vi "Aux2 FPGA.vi"() -> ()   [LabVIEW 2020]
uses:
  <vilib>/LabVIEW Targets/FPGA/cRIO/shared/nicrio_ModuleControls/nicrio_cRIO-9467_Latitude.ctl
  <vilib>/LabVIEW Targets/FPGA/cRIO/shared/nicrio_ModuleControls/nicrio_cRIO-9467_Longitude.ctl
  <vilib>/LabVIEW Targets/FPGA/cRIO/shared/nicrio_ModuleControls/nicrio_cRIO-9467_Altitude.ctl
  <vilib>/rvi/Emulation/niFpgaGetClockAttributes.vi
  <vilib>/rvi/Emulation/niFpgaSctlEmulationGetInTimedLoop.vi
  <vilib>/rvi/Emulation/niFpgaEmulationReportErrorSimple.vi
  subVIs/Front Panel Globals.vi
  <vilib>/rvi/interface/RandomDataEmulation/niFpgaRandomDataHandleErrors.vi
  <vilib>/rvi/Emulation/niFpgaCriticalErrorInLSC.vi
  <vilib>/rvi/Emulation/niFpgaProcessEmulError.vi
  <vilib>/rvi/DataTransferAndStorage/Container/XNode/niFpgaContainer.xnode
  <vilib>/rvi/interface/RandomDataEmulation/nirviRandomDataFpgaReadWriteTemplate.vi
panel:
  out "GPS Self-Survey Complete":bool
  out "GPS Firmware Version":u32
  out "GPS Vendor ID":u16
  out "GPS Altitude (m)":T1 format="%.2f"
  out "GPS Longitude (°)":T2 format="%.6g"
  out "GPS Latitude (°)":T3 format="%.6f"
  out "GPS Serial Number":u32
  out "GPS Time Lock":bool
  out "GPS Time (ns)":u64
  out "GPS Status":T4(ring)
  out "GPS Time Offset":i32
  out "GPS Antenna Status":T5(ring)
  out "GPS Satelites Available":u8
  out "GPS UTC Offset":i8
  out "GPS UTC Offset Valid":bool
  out "Analog Acquisition Looprate":sgl
  in  "Enable Analog Acquisition":bool
  out "Analog Channel Count":i32
  in  "Analog Acquisition Rate":sgl=10000.0
  in  "FPGA USER1 LED":bool
  out "Watchdog Whack Count":u32
  in  "FPGA System Reset":bool
  out "Watchdog ms Since Whack":u32
  in  "Watchdog Whack":bool
  in  "Watchdog Timeout (ms)":u32=3600000
  in  "Watchdog Enable":bool
  out "FPGA Nanosecond Counter":i64
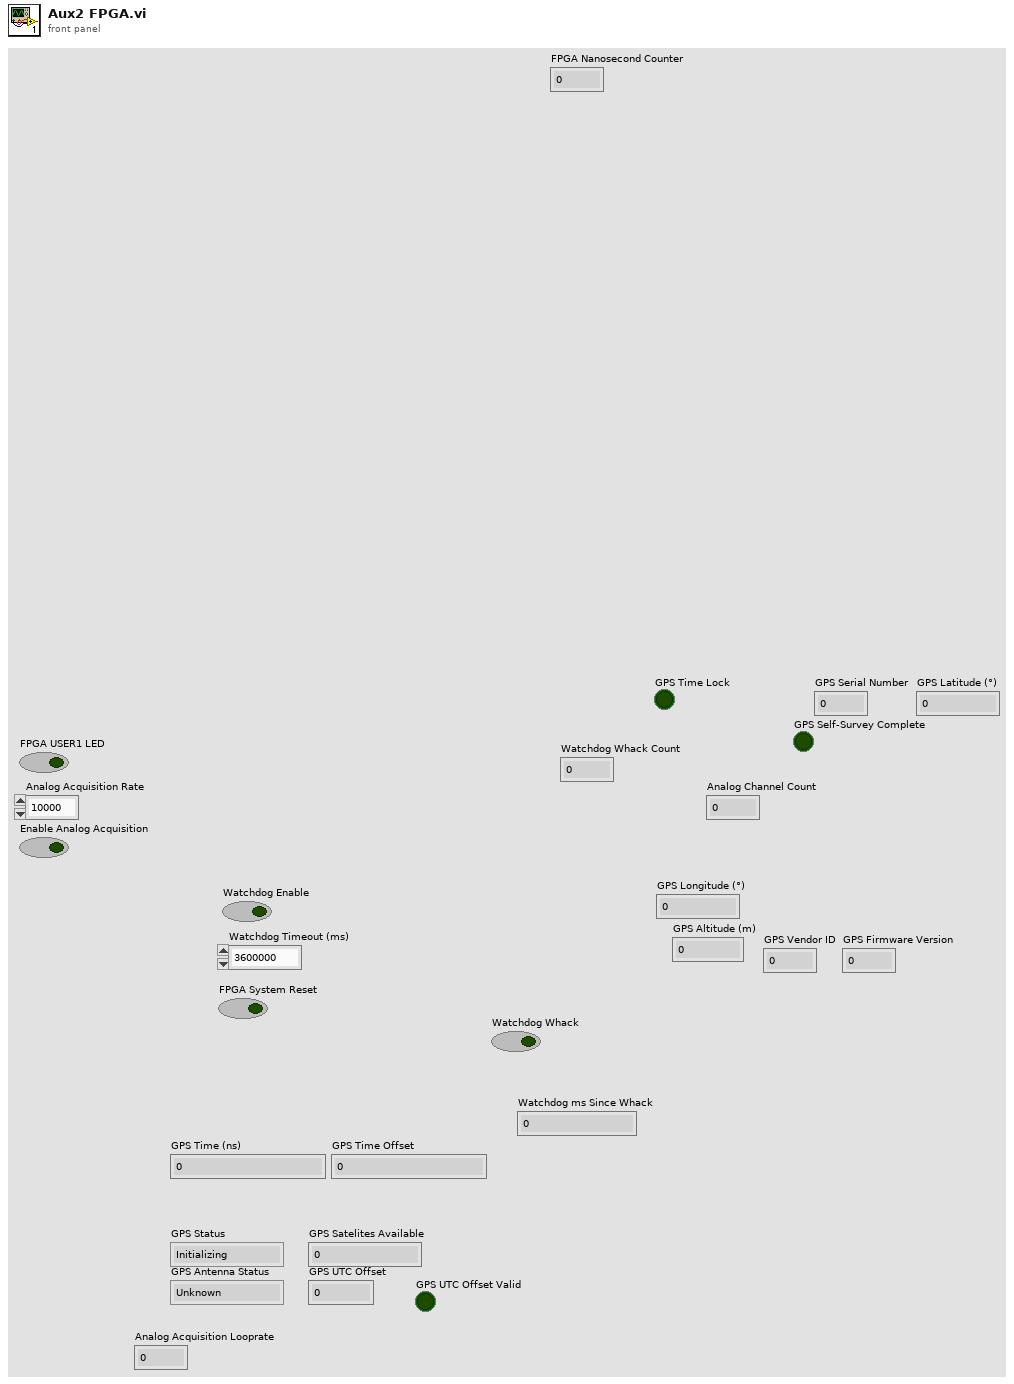
[diagram p1: front panel]
types:
  T1 = typedef "nicrio_cRIO-9467_Altitude.ctl" = fxp<+/-,24,17>
  T2 = typedef "nicrio_cRIO-9467_Longitude.ctl" = fxp<+/-,29,9>
  T3 = typedef "nicrio_cRIO-9467_Latitude.ctl" = fxp<+/-,28,8>
  T4 = enum8{"Initializing", "Normal", "Unable to get fix"}
  T5 = enum8{"Unknown", "Normal", "Absent", "Overcurrent"}
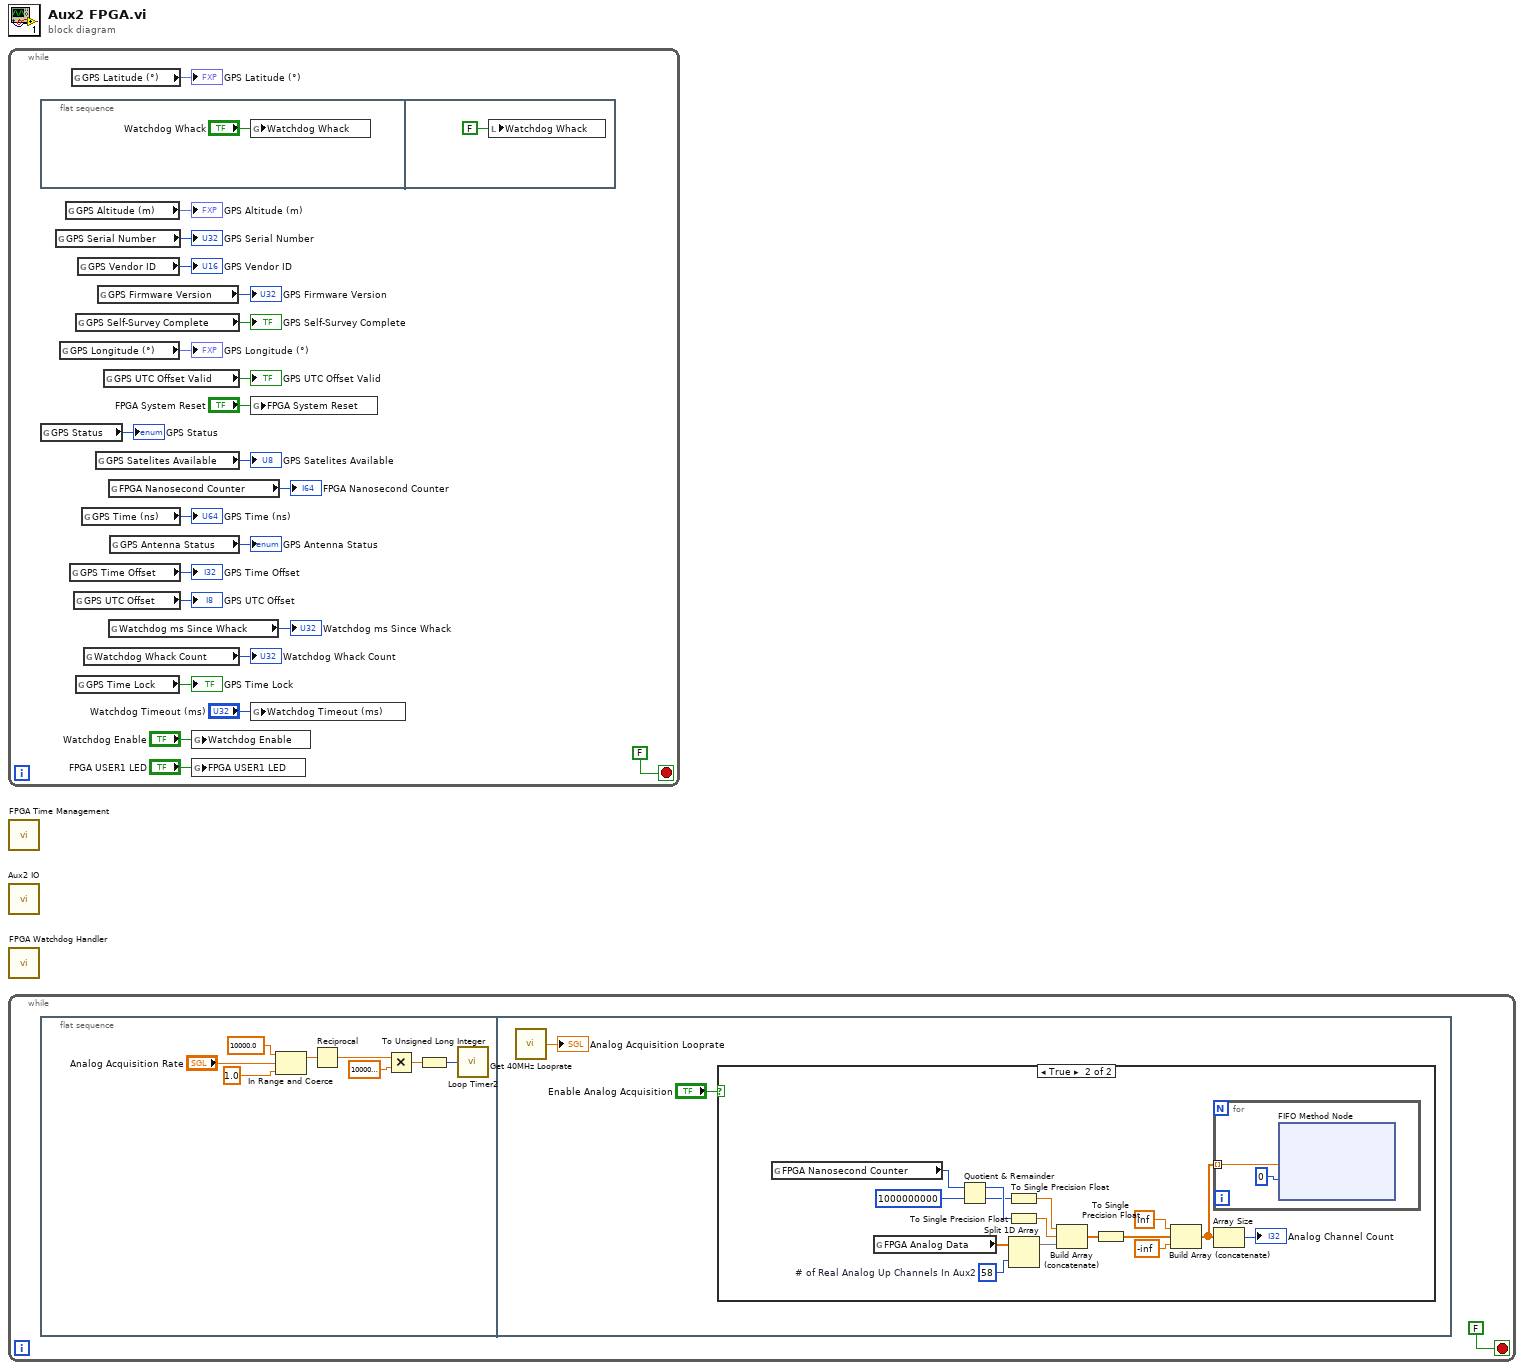
[diagram p0: block diagram]
diagram:
  n1 = while {
    stop <- FALSE stop-if-true
    n2 = flat-sequence {
      frame #0 {
        n3 = global write "Front Panel Globals.vi" "Watchdog Whack"("Watchdog Whack") -> ()
      }
      frame #1 {
        n4 = local write "Watchdog Whack"(FALSE ("Watchdog Enable")) -> ()
      }
    }
    n5 = global read "Front Panel Globals.vi" "GPS Status"() -> (→"GPS Status":T4)
    n6 = global read "Front Panel Globals.vi" "GPS Serial Number"() -> (→"GPS Serial Number":u32)
    n7 = global read "Front Panel Globals.vi" "GPS Longitude (°)"() -> (→"GPS Longitude (°)":T2)
    n8 = global read "Front Panel Globals.vi" "GPS Altitude (m)"() -> (→"GPS Altitude (m)":T1)
    n9 = global read "Front Panel Globals.vi" "GPS Time Offset"() -> (→"GPS Time Offset":i32)
    n10 = global read "Front Panel Globals.vi" "GPS Latitude (°)"() -> (→"GPS Latitude (°)":T3)
    n11 = global read "Front Panel Globals.vi" "GPS UTC Offset"() -> (→"GPS UTC Offset":i8)
    n12 = global read "Front Panel Globals.vi" "GPS Self-Survey Complete"() -> (→"GPS Self-Survey Complete":bool)
    n13 = global read "Front Panel Globals.vi" "GPS Time Lock"() -> (→"GPS Time Lock":bool)
    n14 = global read "Front Panel Globals.vi" "GPS Vendor ID"() -> (→"GPS Vendor ID":u16)
    n15 = global read "Front Panel Globals.vi" "GPS Time (ns)"() -> (→"GPS Time (ns)":u64)
    n16 = global read "Front Panel Globals.vi" "Watchdog Whack Count"() -> (→"Watchdog Whack Count":u32)
    n17 = global read "Front Panel Globals.vi" "GPS Satelites Available"() -> (→"GPS Satelites Available":u8)
    n18 = global read "Front Panel Globals.vi" "GPS Firmware Version"() -> (→"GPS Firmware Version":u32)
    n19 = global read "Front Panel Globals.vi" "GPS UTC Offset Valid"() -> (→"GPS UTC Offset Valid":bool)
    n20 = global read "Front Panel Globals.vi" "FPGA Nanosecond Counter"() -> (→"FPGA Nanosecond Counter":i64)
    n21 = global read "Front Panel Globals.vi" "Watchdog ms Since Whack"() -> (→"Watchdog ms Since Whack":u32)
    n22 = global read "Front Panel Globals.vi" "GPS Antenna Status"() -> (→"GPS Antenna Status":T5)
    n23 = global write "Front Panel Globals.vi" "Watchdog Enable"("Watchdog Enable") -> ()
    n24 = global write "Front Panel Globals.vi" "FPGA USER1 LED"("FPGA USER1 LED") -> ()
    n25 = global write "Front Panel Globals.vi" "FPGA System Reset"("FPGA System Reset") -> ()
    n26 = global write "Front Panel Globals.vi" "Watchdog Timeout (ms)"("Watchdog Timeout (ms)") -> ()
  }
  n27 = call "FPGA Time Management.vi"() -> ()  [unwired: 12 in]
  n28 = call "Aux2 IO.vi"() -> ()  [unwired: 12 in]
  n29 = call "FPGA Watchdog Handler.vi"() -> ()  [unwired: 12 in]
  n30 = while {
    stop <- FALSE stop-if-true
    n31 = flat-sequence {
      frame #0 {
        n32 = In Range and Coerce(upper limit=sgl 10000.0, x="Analog Acquisition Rate", lower limit=sgl 1.0) -> (coerced(x)=w31:sgl)  [unwired: 1 out]
        n33 = Reciprocal(x=w31) -> (1/x=w32:sgl)
        n34 = Multiply(x=w32, y=sgl 1000000.0 ("upper limit")) -> (x*y=w33:sgl)
        n35 = To Unsigned Long Integer(number=w33) -> (unsigned 32bit integer=w34:u32)
        n36 = call "Loop Timer2"("Count(uSec)"=w34) -> ()  [unwired: 1 out]
      }
      frame #1 {
        n37 = call "Get 40MHz Looprate.vi"() -> ("Looprate"=→"Analog Acquisition Looprate":sgl)  [unwired: 5 in]
        n38 = case shown="True" "Enable Analog Acquisition" {
          frame False {
          }
          frame True {
            w37 = 58  # # of Real Analog Up Channels In Aux2
            n39 = global read "Front Panel Globals.vi" "FPGA Nanosecond Counter"() -> (w44:i64)
            n40 = global read "Front Panel Globals.vi" "FPGA Analog Data"() -> (w40:sgl[])
            n41 = Quotient & Remainder(x=w44, y=i64 1000000000) -> (x-y*floor(x/y)=w47:i64, floor(x/y)=w46:i64)
            n42 = To Single Precision Float(number=w46) -> (single precision float=w42:sgl)
            n43 = To Single Precision Float(number=w47) -> (single precision float=w41:sgl)
            n44 = Split 1D Array(array=w40, index=w37) -> (first subarray=w39:sgl[])  [unwired: 1 out]
            n45 = Build Array (concatenate)(w42, w41, w39) -> (w49:sgl[])
            n46 = To Single Precision Float(number=w49) -> (single precision float=w43:sgl[])
            n47 = Build Array (concatenate)(sgl inf ("Mod1/CH3"), w43, sgl -inf ("Mod1/CH3")) -> (w38:sgl[])
            n48 = for {
              tunnel: w38 -> [w53] mode=indexing
              n49 = xnode ("FIFO Method Node")("Element"=w53, "Timeout"=0) -> ()  [unwired: 1 in, 2 out]
            }
            n50 = Array Size(array=w38) -> (size(s)=→"Analog Channel Count":i32)
          }
        }
      }
    }
  }
